vi "Ballard - Arinc-429 - Parameter Page.vi"(8 "error in (no error)":errorcluster, 11 "Node Ptr":T3 format="%.0x") -> (0 "error out":errorcluster)   [LabVIEW 2017, in "Ballard Arinc-429 System Explorer.lvlib"]
uses:
  Ballard Arinc-429 System Explorer.lvlib
  <vilib>/NI Veristand/Custom Device API/Custom Device Item Ref.ctl
  Shared/Controls and Global/Start Bit.ctl
  Shared/Controls and Global/Number of Bits.ctl
  Shared/Controls and Global/Global.vi
  <vilib>/NI Veristand/Custom Device API/Get Item Property (U32).vi
  <vilib>/NI Veristand/Custom Device API/Get Item Property (Boolean).vi
  <vilib>/NI Veristand/Custom Device API/Get Item Property (Double).vi
  <vilib>/NI Veristand/Custom Device API/Get Item Property (I32).vi
  <vilib>/NI Veristand/Custom Device API/Set Item Property (I32).vi
  <vilib>/NI Veristand/Custom Device API/Set Item Property (Boolean).vi
  <vilib>/NI Veristand/Custom Device API/Set Item Property (Double).vi
  <vilib>/NI Veristand/Custom Device API/Set Item Property (U32).vi
  <vilib>/NI Veristand/Custom Device API/Custom Device API.lvlib
  Shared/Ballard Arinc-429 Shared.lvlib
panel:
  out "Default Value (Raw Bits)":u32
  out "TiggerDValChange":bool
  in  "Scale Offset":dbl format="%#_6f"
  in  "Scale Factor":dbl format="%#_6f"
  in  "Signed?":bool
  out "Default Value (Scaled)":dbl
  in  "Number of Bits":T1=1 min=1 max=32
  in  "Start Bit":T2=1
  in  "Header":cluster{"Section Name":string}={"Section Name"="Ballard 429 Parameter"}
  in  "Description":string
  in  "Name":string
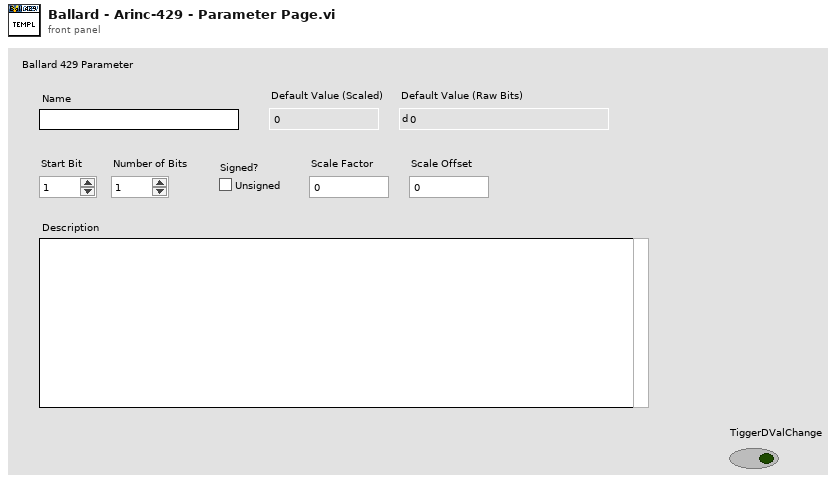
[diagram p1: front panel]
types:
  T1 = typedef "Ballard Arinc-429 Shared.lvlib/Number of Bits.ctl" = i32
  T2 = typedef "Ballard Arinc-429 Shared.lvlib/Start Bit.ctl" = i32
  T3 = typedef "Custom Device API.lvlib/Custom Device Item Ref.ctl" = u64
  T4 = typedef "Custom Device API.lvlib/Custom Device Item Info.ctl" = cluster{"Name":string, "Is Channel":bool, "GUID":string, "Is Waveform":bool}
  T5 = typedef "Custom Device API.lvlib/Custom Device Channel.ctl" = cluster{"Type":T6, "Units":string, "Default Value":dbl, "Faultable":bool, "Scalable":bool}
  T6 = typedef "Custom Device API.lvlib/Custom Device Channel Type.ctl" = enum16{"Input", "Output"}
  T7 = typedef "Custom Device API.lvlib/Custom Device Commands.ctl" = enum16{"Default", "Item renamed", "Shutdown", "Dynamic button pressed"}
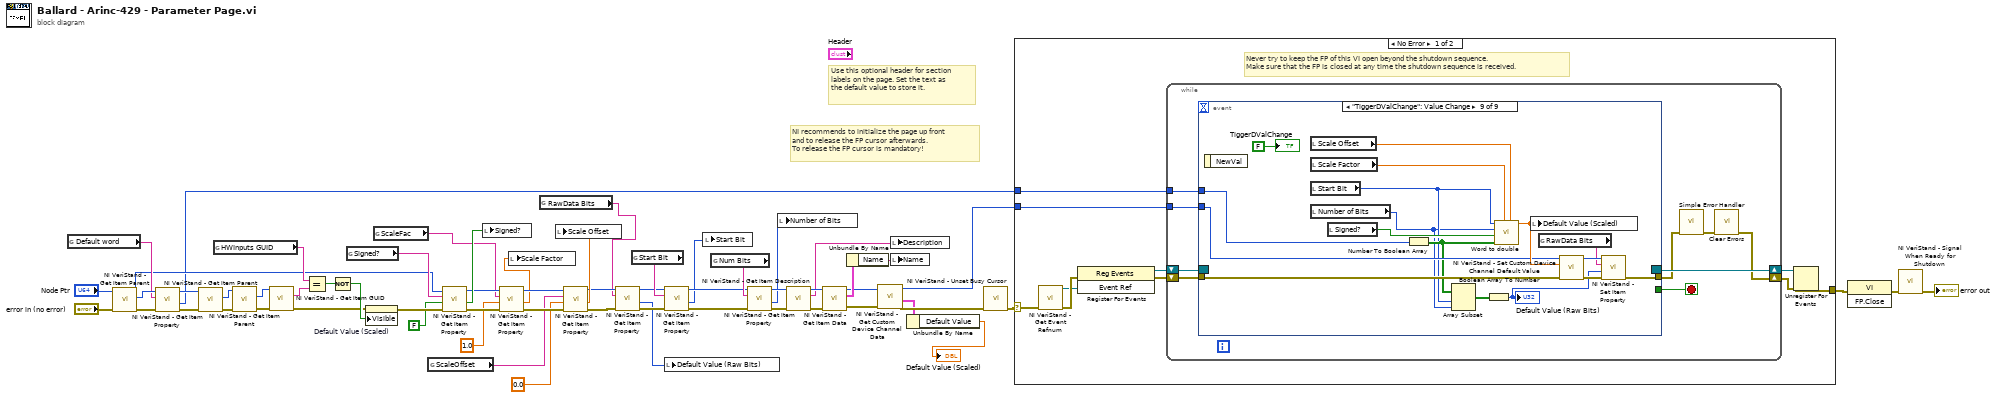
[diagram p0: block diagram]
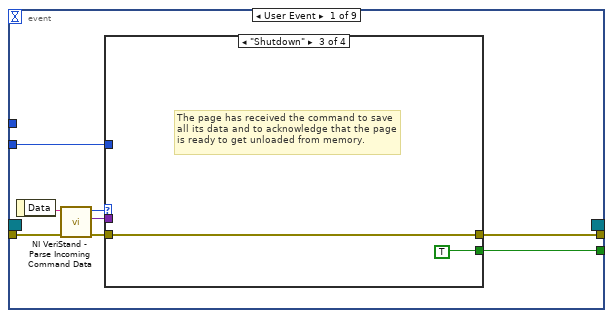
[diagram p2: hidden frame]
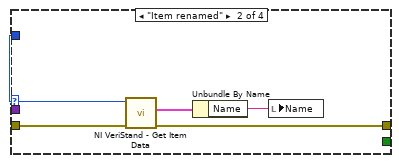
[diagram p4: hidden frame]
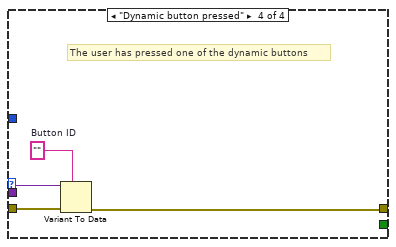
[diagram p5: hidden frame]
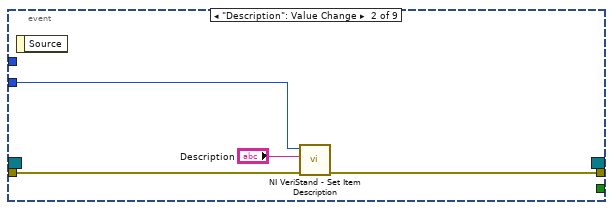
[diagram p6: hidden frame]
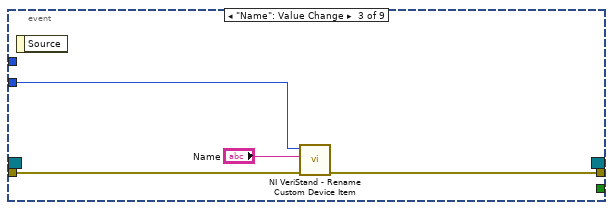
[diagram p7: hidden frame]
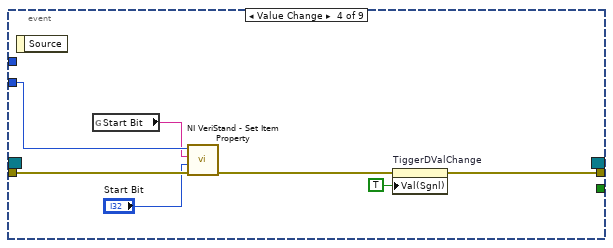
[diagram p8: hidden frame]
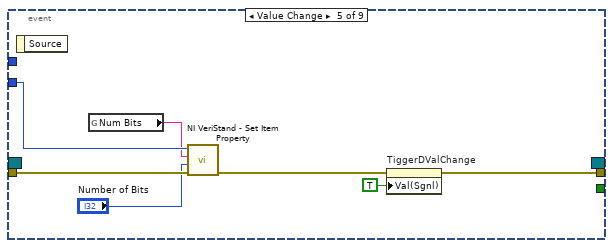
[diagram p9: hidden frame]
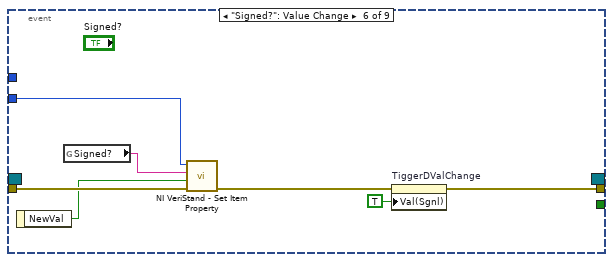
[diagram p10: hidden frame]
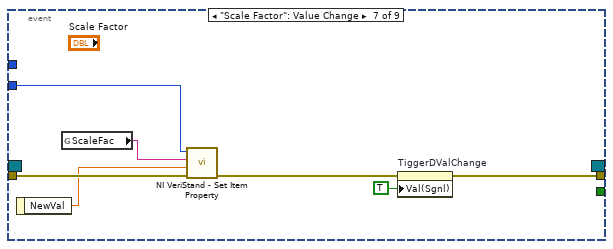
[diagram p11: hidden frame]
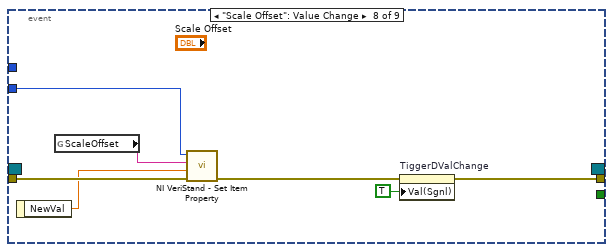
[diagram p12: hidden frame]
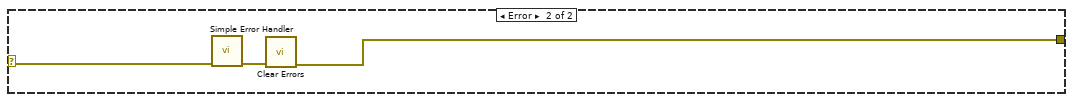
[diagram p13: hidden frame]
diagram:
  # "Use this optional header for section labels on the page. Set the text as the default value to store it."
  # "NI recommends to initialize the page up front\nand to release the FP cursor afterwards.\nTo release the FP cursor is mandatory!"
  n1 = global read "Global.vi" "Default word"() -> (w27:string)
  n2 = call <vilib>:"NI VeriStand - Get Item Parent.vi"("error in (no error)"="error in (no error)", "Item Ref in"="Node Ptr") -> ("error out"=w30:errorcluster, "Parent Ref"=w29:T3, "Item Ref out"=w12:T3)  [unwired: 6 in, 1 out]
  n3 = call-poly <vilib>:"NI VeriStand - Get Item Property.vi"("error in (no error)"=w30, "Property Name"=w27, "Item Ref in"=w29) -> ("error out"=w26:errorcluster, "Value"=w9:u32, "Item Ref out"=w28:T3)  [unwired: 5 in, 1 out]
  n4 = call <vilib>:"NI VeriStand - Get Item Parent.vi"("error in (no error)"=w26, "Item Ref in"=w28) -> ("error out"=w33:errorcluster, "Parent Ref"=w32:T3)  [unwired: 6 in, 2 out]
  n5 = global read "Global.vi" "HWInputs GUID"() -> (w41:string)
  n6 = call <vilib>:"NI VeriStand - Get Item Parent.vi"("error in (no error)"=w33, "Item Ref in"=w32) -> ("error out"=w44:errorcluster, "Parent Ref"=w43:T3)  [unwired: 6 in, 2 out]
  n7 = call <vilib>:"NI VeriStand - Get Item GUID.vi"("error in (no error)"=w44, "Item Ref in"=w43) -> ("error out"=w25:errorcluster, "GUID"=w42:string)  [unwired: 7 in, 1 out]
  n8 = Equal?(x=w41, y=w42) -> (x = y?=w35:bool)
  n9 = Not(x=w35) -> (.not. x?=w34:bool)
  n10 = global read "Global.vi" "Signed?"() -> (w23:string)
  n11 = property on="Default Value (Scaled)" class="DigNum (strict)"(error in=w25, "Visible"=w34) -> (error out=w24:errorcluster)  [unwired: 1 in, 1 out]
  n12 = global read "Global.vi" "ScaleFac"() -> (w18:string)
  n13 = global read "Global.vi" "ScaleOffset"() -> (w14:string)
  n14 = call-poly <vilib>:"NI VeriStand - Get Item Property.vi"("error in (no error)"=w24, "Default Value"=FALSE, "Property Name"=w23, "Item Ref in"=w12) -> ("error out"=w20:errorcluster, "Value"=w21:bool, "Item Ref out"=w19:T3)  [unwired: 4 in, 1 out]
  n15 = local write "Signed?"(w21) -> ()
  n16 = call-poly <vilib>:"NI VeriStand - Get Item Property.vi"("error in (no error)"=w20, "Default Value"=1.0 ("Scale Factor"), "Property Name"=w18, "Item Ref in"=w19) -> ("error out"=w16:errorcluster, "Value"=w10:dbl, "Item Ref out"=w15:T3)  [unwired: 4 in, 1 out]
  n17 = local write "Scale Factor"(w10) -> ()
  n18 = global read "Global.vi" "RawData Bits"() -> (w2:string)
  n19 = call-poly <vilib>:"NI VeriStand - Get Item Property.vi"("error in (no error)"=w16, "Default Value"=0.0 ("Scale Factor"), "Property Name"=w14, "Item Ref in"=w15) -> ("error out"=w5:errorcluster, "Value"=w11:dbl, "Item Ref out"=w6:T3)  [unwired: 4 in, 1 out]
  n20 = local write "Scale Offset"(w11) -> ()
  n21 = call-poly <vilib>:"NI VeriStand - Get Item Property.vi"("error in (no error)"=w5, "Property Name"=w2, "Item Ref in"=w6) -> ("error out"=w3:errorcluster, "Value"=w1:u32, "Item Ref out"=w4:T3)  [unwired: 5 in, 1 out]
  n22 = global read "Global.vi" "Start Bit"() -> (w49:string)
  n23 = local write "Default Value (Raw Bits)"(w1) -> ()
  n24 = call-poly <vilib>:"NI VeriStand - Get Item Property.vi"("error in (no error)"=w3, "Property Name"=w49, "Item Ref in"=w4) -> ("error out"=w47:errorcluster, "Value"=w7:i32, "Item Ref out"=w48:T3)  [unwired: 5 in, 1 out]
  n25 = local write "Start Bit"(w7) -> ()
  n26 = global read "Global.vi" "Num Bits"() -> (w52:string)
  n27 = call-poly <vilib>:"NI VeriStand - Get Item Property.vi"("error in (no error)"=w47, "Property Name"=w52, "Item Ref in"=w48) -> ("error out"=w50:errorcluster, "Value"=w8:i32, "Item Ref out"=w51:T3)  [unwired: 5 in, 1 out]
  n28 = local write "Number of Bits"(w8) -> ()
  n29 = call <vilib>:"NI VeriStand - Get Item Description.vi"("error in (no error)"=w50, "Item Ref in"=w51) -> ("error out"=w55:errorcluster, "Description"=w56:string, "Item Ref out"=w57:T3)  [unwired: 7 out]
  n30 = call <vilib>:"NI VeriStand - Get Item Data.vi"("error in (no error)"=w55, "Item Ref in"=w57) -> ("error out"=w40:errorcluster, "Item Info"=w54:T4, "Item Ref out"=w39:T3)  [unwired: 7 out]
  n31 = Unbundle By Name(w54) -> ("Name"=w53:string)
  n32 = call <vilib>:"NI VeriStand - Get Custom Device Channel Data.vi"("error in (no error)"=w40, "Channel Ref in"=w39) -> ("error out"=w37:errorcluster, "Channel"=w36:T5, "Channel Ref out"=w38:T3)  [unwired: 4 in, 3 out]
  n33 = local write "Description"(w56) -> ()
  n34 = local write "Name"(w53) -> ()
  n35 = Unbundle By Name(w36) -> ("Default Value"=→"Default Value (Scaled)":dbl)
  n36 = call <vilib>:"NI VeriStand - Unset Busy Cursor.vi"("error in (no error)"=w37) -> ("error out"=w58:errorcluster)  [unwired: 10 out]
  n37 = case shown="No Error" w58 {
    selector: w58 -> [w63 w163]
    tunnel: [w68 w161] -> w61
    tunnel: w38 -> [w64 _]
    tunnel: w9 -> [w62 _]
    frame No Error {
      # "Never try to keep the FP of this VI open beyond the shutdown sequence.\nMake sure that the FP is closed at any time the shutdown sequence is received."
      n38 = call <vilib>:"NI VeriStand - Get Event Refnum.vi"("error in (no error)"=w63) -> ("error out"=w71:errorcluster, "Event Ref"=w67:refnum<user-event>)  [unwired: 9 out]
      n39 = register-events(error in=w71, w67) -> (reference out=w65:refnum<event-registration>, error out=w66:errorcluster)  [unwired: 1 in]
      n40 = while {
        tunnel: w64 -> [w76]
        shift-right: [w73] -> w69
        shift-left: w66 -> [w79]
        shift-right: [w80] -> w70
        shift-left: w65 -> [w78]
        tunnel: w62 -> [w72]
        stop <- w77 stop-if-true
        n41 = event shown="[8] \"TiggerDValChange\": Value Change" {
          selector: w78 -> [_ _ _ _ _ _ _ _ _]
          dyn-events: [_ _ _ _ _ _ _ _ _] -> w80
          timeout: _ -> [_ _ _ _ _ _ _ _ _]
          tunnel: w79 -> [w88 w103 w107 w115 w122 w129 w136 w143 w160]
          tunnel: [w84 _ _ _ _ _ _ _ _] -> w77
          tunnel: [w83 w102 w106 w110 w116 w123 w130 w137 w146] -> w75
          tunnel: w76 -> [w82 w104 w108 w114 w121 w128 w135 w142 w158]
          tunnel: w72 -> [_ _ _ _ _ _ _ _ w157]
          event User Event {
            n42 = event-data() -> ("Data"=w87:string)  [unwired: 1 out]
            n43 = call <vilib>:"NI VeriStand - Parse Incoming Command Data.vi"("error in (no error)"=w88, "Incoming data"=w87) -> ("error out"=w86:errorcluster, "Outgoing data"=w81:variant, "Action"=w85:T7)  [unwired: 7 out]
            n44 = case shown="\"Shutdown\"" w85 {
              tunnel: w86 -> [w89 w94 w95 w100]
              tunnel: [_ _ TRUE _] -> w84
              tunnel: [w89 w91 w95 w97] -> w83
              tunnel: w82 -> [_ w93 _ _]
              tunnel: w81 -> [_ _ _ w99]
              frame "Default", Default {
              }
              frame "Item renamed" {
                n45 = call <vilib>:"NI VeriStand - Get Item Data.vi"("error in (no error)"=w94, "Item Ref in"=w93) -> ("error out"=w91:errorcluster, "Item Info"=w92:T4)  [unwired: 8 out]
                n46 = Unbundle By Name(w92) -> ("Name"=w90:string)
                n47 = local write "Name"(w90) -> ()
              }
              frame "Shutdown" {
                # "The page has received the command to save all its data and to acknowledge that the page is ready to get unloaded from memory."
              }
              frame "Dynamic button pressed" {
                w98 = ""  # Button ID
                # "The user has pressed one of the dynamic buttons"
                n48 = Variant To Data(error in=w100, type=w98, Variant=w99) -> (error out=w97:errorcluster)  [unwired: 1 out]
              }
            }
          }
          event "Description": Value Change {
            n49 = event-data() -> ()  [unwired: 2 out]
            n50 = call <vilib>:"NI VeriStand - Set Item Description.vi"("error in (no error)"=w103, "Description"="Description", "Item Ref in"=w104) -> ("error out"=w102:errorcluster)  [unwired: 8 out]
          }
          event "Name": Value Change {
            n51 = event-data() -> ()  [unwired: 2 out]
            n52 = call <vilib>:"NI VeriStand - Rename Custom Device Item.vi"("error in (no error)"=w107, "New Name"="Name", "Item Ref in"=w108) -> ("error out"=w106:errorcluster)  [unwired: 6 in, 2 out]
          }
          event Value Change {
            n53 = event-data() -> ()  [unwired: 2 out]
            n54 = global read "Global.vi" "Start Bit"() -> (w113:string)
            n55 = call-poly <vilib>:"NI VeriStand - Set Item Property.vi"("error in (no error)"=w115, "Value"="Start Bit", "Property Name"=w113, "Item Ref in"=w114) -> ("error out"=w111:errorcluster)  [unwired: 5 in, 2 out]
            n56 = property on="TiggerDValChange" class="Bool (strict)"(error in=w111, "Val(Sgnl)"=TRUE ("Value (Signaling)")) -> (error out=w110:errorcluster)  [unwired: 1 in, 1 out]
          }
          event Value Change {
            n57 = event-data() -> ()  [unwired: 2 out]
            n58 = global read "Global.vi" "Num Bits"() -> (w120:string)
            n59 = call-poly <vilib>:"NI VeriStand - Set Item Property.vi"("error in (no error)"=w122, "Value"="Number of Bits", "Property Name"=w120, "Item Ref in"=w121) -> ("error out"=w117:errorcluster)  [unwired: 5 in, 2 out]
            n60 = property on="TiggerDValChange" class="Bool (strict)"(error in=w117, "Val(Sgnl)"=TRUE ("Value (Signaling)")) -> (error out=w116:errorcluster)  [unwired: 1 in, 1 out]
          }
          event "Signed?": Value Change {
            n61 = event-data() -> ("NewVal"=w126:bool)  [unwired: 1 out]
            n62 = global read "Global.vi" "Signed?"() -> (w127:string)
            n63 = call-poly <vilib>:"NI VeriStand - Set Item Property.vi"("error in (no error)"=w129, "Value"=w126, "Property Name"=w127, "Item Ref in"=w128) -> ("error out"=w124:errorcluster)  [unwired: 5 in, 2 out]
            n64 = property on="TiggerDValChange" class="Bool (strict)"(error in=w124, "Val(Sgnl)"=TRUE ("Value (Signaling)")) -> (error out=w123:errorcluster)  [unwired: 1 in, 1 out]
          }
          event "Scale Factor": Value Change {
            n65 = event-data() -> ("NewVal"=w133:dbl)  [unwired: 1 out]
            n66 = global read "Global.vi" "ScaleFac"() -> (w134:string)
            n67 = call-poly <vilib>:"NI VeriStand - Set Item Property.vi"("error in (no error)"=w136, "Value"=w133, "Property Name"=w134, "Item Ref in"=w135) -> ("error out"=w131:errorcluster)  [unwired: 5 in, 2 out]
            n68 = property on="TiggerDValChange" class="Bool (strict)"(error in=w131, "Val(Sgnl)"=TRUE ("Value (Signaling)")) -> (error out=w130:errorcluster)  [unwired: 1 in, 1 out]
          }
          event "Scale Offset": Value Change {
            n69 = event-data() -> ("NewVal"=w140:dbl)  [unwired: 1 out]
            n70 = global read "Global.vi" "ScaleOffset"() -> (w141:string)
            n71 = call-poly <vilib>:"NI VeriStand - Set Item Property.vi"("error in (no error)"=w143, "Value"=w140, "Property Name"=w141, "Item Ref in"=w142) -> ("error out"=w138:errorcluster)  [unwired: 5 in, 2 out]
            n72 = property on="TiggerDValChange" class="Bool (strict)"(error in=w138, "Val(Sgnl)"=TRUE ("Value (Signaling)")) -> (error out=w137:errorcluster)  [unwired: 1 in, 1 out]
          }
          event "TiggerDValChange": Value Change {
            n73 = event-data() -> ()  [unwired: 2 out]
            n74 = local read "Scale Offset"() -> (w154:dbl)
            n75 = local read "Scale Factor"() -> (w155:dbl)
            n76 = local read "Start Bit"() -> (w151:T2)
            n77 = local read "Number of Bits"() -> (w150:T1)
            n78 = local read "Signed?"() -> (w156:bool)
            n79 = Number To Boolean Array(number=w157) -> (Boolean array=w152:bool[])
            n80 = Array Subset(array=w152, index=w151, length=w150) -> (w149:bool[])
            n81 = Boolean Array To Number(Boolean array=w149) -> (number=w145:u32)
            "Default Value (Raw Bits)" <- w145
            n82 = call "Word to double.vi"("ScaleOffset (0)"=w154, "ScaleFac (1)"=w155, "Word"=w152, "Signed? (F)"=w156, "Number of Bits"=w150, "Start Bit"=w151) -> ("Double"=w159:dbl)  [unwired: 5 in]
            n83 = local write "Default Value (Scaled)"(w159) -> ()
            n84 = global read "Global.vi" "RawData Bits"() -> (w144:string)
            n85 = call <vilib>:"NI VeriStand - Set Custom Device Channel Default Value.vi"("error in (no error)"=w160, "Default Value"=w159, "Channel Ref in"=w158) -> ("error out"=w148:errorcluster, "Channel Ref out"=w147:T3)  [unwired: 7 in]
            n86 = call-poly <vilib>:"NI VeriStand - Set Item Property.vi"("error in (no error)"=w148, "Value"=w145, "Property Name"=w144, "Item Ref in"=w147) -> ("error out"=w146:errorcluster)  [unwired: 5 in, 2 out]
            "TiggerDValChange" <- FALSE
          }
        }
        n87 = call <vilib>:"Simple Error Handler.vi"("error in (no error)"=w75) -> ("error out"=w74:errorcluster)  [unwired: 1 in, 7 out]
        n88 = call <vilib>:"Clear Errors.vi"("error in (no error)"=w74) -> ("error out"=w73:errorcluster)  [unwired: 1 in, 5 out]
      }
      n89 = Unregister For Events(event registration refnum=w70, error in=w69) -> (error out=w68:errorcluster)
    }
    frame Error {
      n90 = call <vilib>:"Simple Error Handler.vi"("error in (no error)"=w163) -> ("error out"=w162:errorcluster)  [unwired: 1 in, 7 out]
      n91 = call <vilib>:"Clear Errors.vi"("error in (no error)"=w162) -> ("error out"=w161:errorcluster)  [unwired: 1 in, 5 out]
    }
  }
  n92 = invoke class="VI" method="FP.Close"(error in=w61) -> (error out=w60:errorcluster)  [unwired: 2 in, 2 out]
  n93 = call <vilib>:"NI VeriStand - Signal When Ready for Shutdown.vi"("error in (no error)"=w60) -> ("error out"=→"error out":errorcluster)  [unwired: 10 out]
